vi "Read Stop.vi"(7 "Actor in":refnum<class "Actor.lvclass">) -> (2 "Stop":bool)   [LabVIEW 2020, in "jettl.lvlib"]
uses:
  jettl.lvlib
  Actor/Actor.lvclass
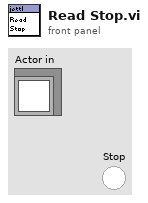
[diagram p1: front panel]
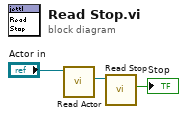
[diagram p0: block diagram]
diagram:
  n1 = call-dynamic "Read Actor.vi"("Actor in"="Actor in") -> ("Actor"=w2:refnum<class "Actor.lvclass">)  [unwired: 10 in]
  n2 = call-dynamic "Read Stop.vi"("Actor in"=w2) -> ("Stop"=→"Stop":bool)  [unwired: 10 in]
